vi "Begin.vi"(8 "error in":errorcluster) -> (0 "error out":errorcluster)   [LabVIEW 2017]
doc: "Called before other user functions, this VI is expected to open initial I/O refnums, load in file data, and do all program initialization. Notice that the <B>error out</B> terminal is simply used for data flow. Wiring it to other structures or subVIs ensures that this VI runs first."
uses:
  <vilib>/Rock Robotics/WPI/DriverStation/WPI_DriverStationRobotMode2.ctl
  <vilib>/Rock Robotics/WPI/Solenoid/WPI_SolenoidChannel.ctl
  <vilib>/Rock Robotics/WPI/ThirdParty/Phoenix-LabVIEW/Motor Controller/Controls/CTRE_Phoenix_MotorControl_NeutralMode.ctl
  <vilib>/Rock Robotics/SystemInterfaces/DIO/FPGA_DIOChannel.ctl
  <vilib>/Rock Robotics/WPI/Joystick/WPI_JoystickDeviceEnum.ctl
  <vilib>/Rock Robotics/WPI/ThirdParty/Phoenix-LabVIEW/Motor Controller/Controls/CTRE_Phoenix_MotorControl_VelocityMeasurementPeriod.ctl
  <vilib>/Rock Robotics/WPI/ThirdParty/Phoenix-LabVIEW/Motor Controller/Controls/CTRE_Phoenix_MotorControl_StatusFrameEnhanced.ctl
  Robot Global Data.vi
  <vilib>/Rock Robotics/WPI/Solenoid/WPI_SolenoidOpenDouble.vi
  <vilib>/Rock Robotics/WPI/Switch/WPI_SwitchOpenLimit.vi
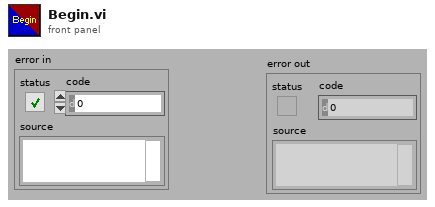
[diagram p1: front panel]
types:
  T1 = typedef "WPI_DriverStationRobotMode2.ctl" = enum16{"Autonomous Disabled", "Autonomous Enabled", "Teleop Disabled", "Teleop Enabled", "Disconnected", "Finish", "Test Disabled", "Test Enabled", "Emergency Stopped"}
  T2 = enum16{"Manual", "Turn For Angle", "Drive For Distance", "Motion Profile", "Recorded Auto File"}
  T3 = typedef "WPI_JoystickDeviceEnum.ctl" = enum16{"USB 0", "USB 1", "USB 2", "USB 3", "USB 4", "USB 5"}
  T4 = typedef "WPI_SolenoidChannel.ctl" = enum8{"Solenoid 0", "Solenoid 1", "Solenoid 2", "Solenoid 3", "Solenoid 4", "Solenoid 5", "Solenoid 6", "Solenoid 7", "Invalid"}
  T5 = typedef "CTRE_Phoenix_MotorControl_StatusFrameEnhanced.ctl" = u16
  T6 = typedef "CTRE_Phoenix_MotorControl_VelocityMeasurementPeriod.ctl" = u16
  T7 = typedef "WPI_MotorControlDeviceRef.ctl" = cluster{"DeviceStatus":errorcluster, "Type":T8, "PWM":cluster{"PWM Channel":T9, "DeadBand":T10}, "CAN":cluster{"Device Number":u8, "SetOutput VI Ref":variant, "GetOutput VI Ref":variant, "Enable VI Ref":variant, "Disable VI Ref":variant, "Data":variant}, "Invert":bool, "DIO PWM":cluster{"PWM \"Enable\" Channel":T9, "DIOChannel":T11, "PWM Rate":dbl}}
  T8 = typedef "WPI_MotorControlType.ctl" = enum16{"PWM", "CAN", "DIO PWM"}
  T9 = typedef "FPGA_DIOPWMChannel.ctl" = enum8{"PWM 0", "PWM 1", "PWM 2", "PWM 3", "PWM 4", "PWM 5", "PWM 6", "PWM 7", "PWM 8", "PWM 9", "PWM MXP 0", "PWM MXP 1", "PWM MXP 2", "PWM MXP 3", "PWM MXP 4", "PWM MXP 5", "PWM MXP 6", "PWM MXP 7", "PWM MXP 8", "PWM MXP 9", "Invalid"}
  T10 = typedef "WPI_PWMDeadband.ctl" = cluster{"Name":string, "maxPositivePwm":i32, "minPositivePwm":i32, "centerPwm":i32, "maxNegativePwm":i32, "minNegativePwm":i32, "angularRange":u16}
  T11 = typedef "FPGA_DIOChannel.ctl" = enum8{"DIO 0", "DIO 1", "DIO 2", "DIO 3", "DIO 4", "DIO 5", "DIO 6", "DIO 7", "DIO 8", "DIO 9", "DIO MXP 0", "DIO MXP 1", "DIO MXP 2", "DIO MXP 3", "DIO MXP 4", "DIO MXP 5", "DIO MXP 6", "DIO MXP 7", "DIO MXP 8", "DIO MXP 9", "DIO MXP 10", "DIO MXP 11", "DIO MXP 12", "DIO MXP 13", "DIO MXP 14", "DIO MXP 15", "SPI Port CS1", "SPI Port CS2", "SPI Port CS3", "SPI Port MISO", "SPI Port MOSI", "Invalid"}
  T12 = typedef "WPI_JoystickDevRef.ctl" = cluster{"Device":T3}
  T13 = typedef "WPI_SolenoidDevRef.ctl" = cluster{"DevStatus":errorcluster, "Pneumatics Control Module":u8, "Forward Solenoid Channel":T4, "Reverse Solenoid Channel":T4}
  T14 = typedef "CTRE_Phoenix_MotorControl_NeutralMode.ctl" = enum8{"EEPROMSetting", "Override to Coast", "Override to Brake"}
  T15 = typedef "WPI_SwitchDevRef.ctl" = cluster{"DevStatus":errorcluster, "DIO Channel":T11, "CntIndex":T16, "Normally Closed":bool}
  T16 = typedef "FPGA_CounterCtrSystemIndex.ctl" = enum8{"Ctr 0", "Ctr 1", "Ctr 2", "Ctr 3", "Ctr 4", "Ctr 5", "Ctr 6", "Ctr 7", "Invalid"}
  T17 = typedef "WPI_CompressorDevRef.ctl" = cluster{"DevStatus":errorcluster, "Pneumatics Control Module":u8}
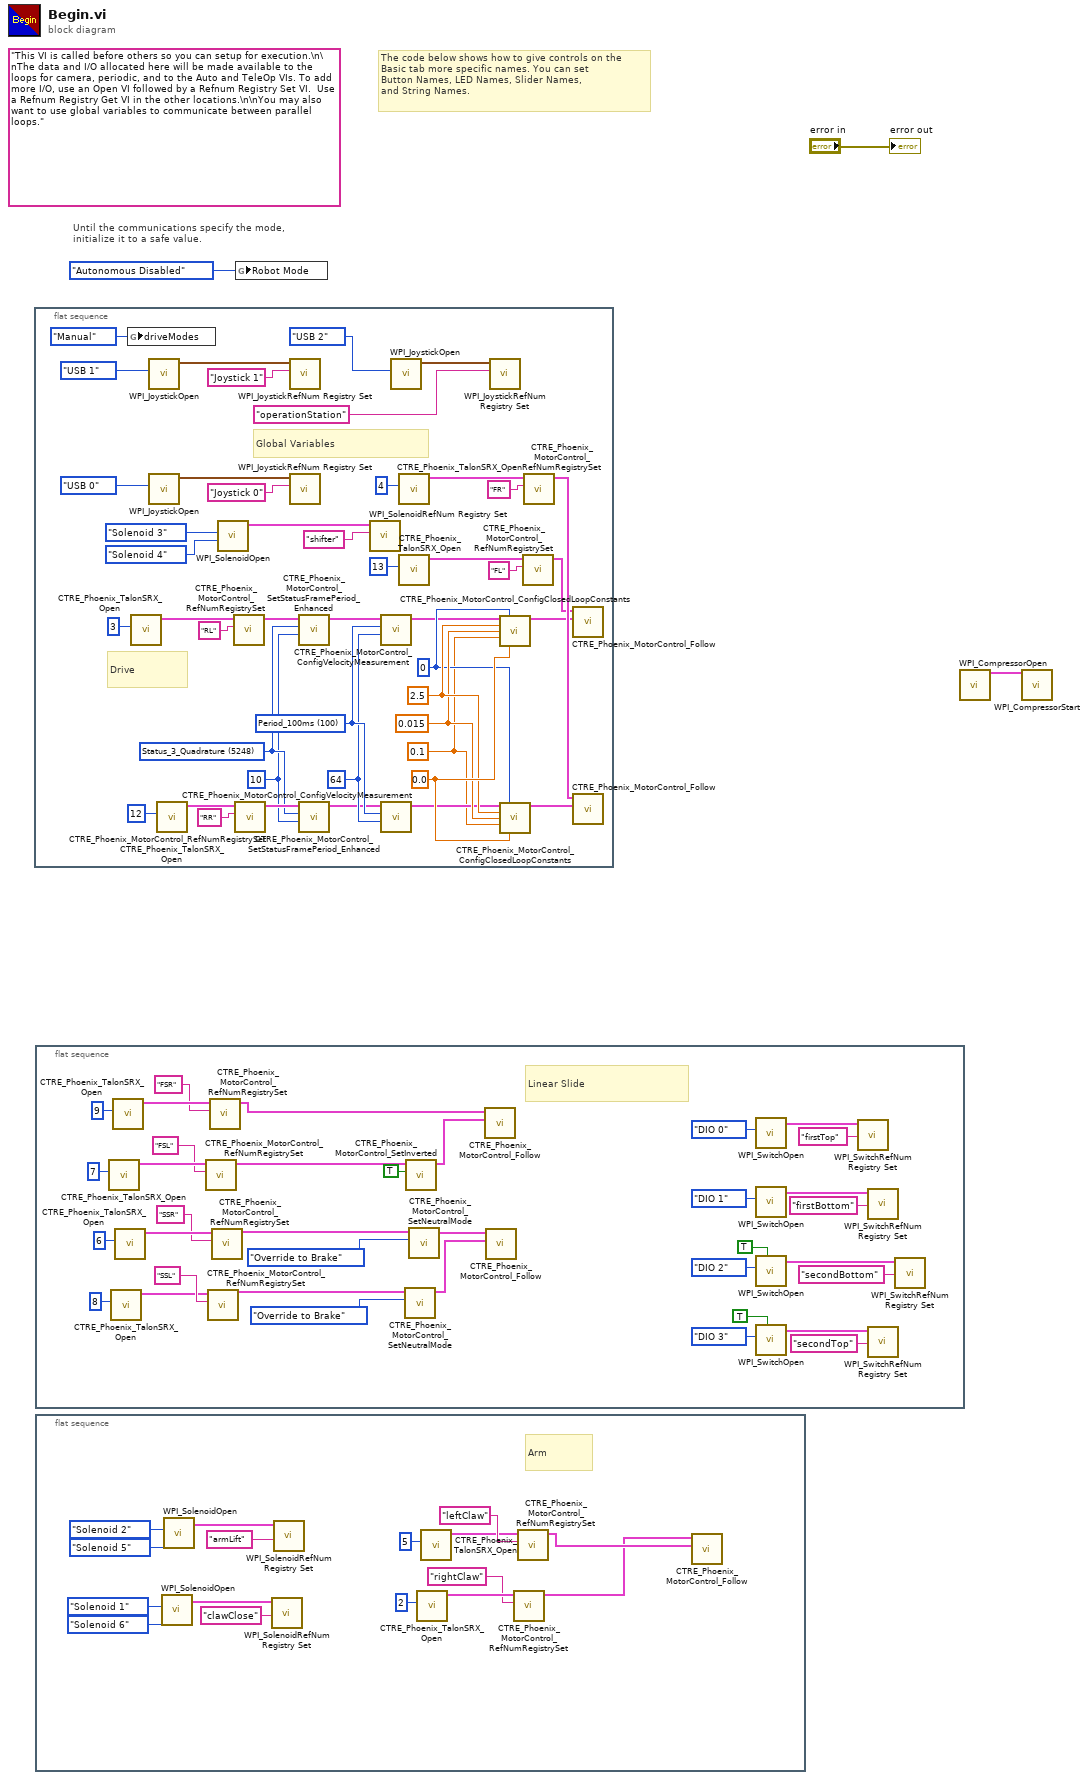
[diagram p0: block diagram]
diagram:
  (unwired) "This VI is called before others so you can setup for execution.\n\nThe data and I/O allocated here will be made available to the loops for camera, periodic, and to the Auto and TeleOp VIs. To add more I/O, use an Open VI followed by a Refnum Registry Set VI.  Use a Refnum Registry Get VI in the other locations.\n\nYou may also want to use global variables to communicate between parallel loops."
  # "The code below shows how to give controls on the\nBasic tab more specific names. You can set\nButton Names, LED Names, Slider Names,\nand String Names."
  # "Until the communications specify the mode,\ninitialize it to a safe value."
  n1 = flat-sequence {
    frame #0 {
      w4 = 10 ("periodMs")
      w5 = T5 5248 items=["Status_1_General"=5120, "Status_2_Feedback0"=5184, "Status_3_Quadrature"=5248, "Status_4_AinTempVbat"=5312, "Status_6_Misc"=5440, "Status_7_CommStatus"=5504, "Status_8_PulseWidth"=5568, "Status_9_MotProfBuffer"=5632, "Status_10_MotionMagic"=5696, "Status_11_UartGadgeteer"=5760, "Status_12_Feedback1"=5824, "Status_13_Base_PIDF0"=5888, "Status_14_Turn_PIDF1"=5952, "Status_15_FirmwareApiStatus"=6016] ("Status Frame")
      w11 = 0.1 ("D")
      w12 = 64 ("Window Size")
      w13 = T6 100 items=["Period_1ms"=1, "Period_2ms"=2, "Period_5ms"=5, "Period_10ms"=10, "Period_20ms"=20, "Period_25ms"=25, "Period_50ms"=50, "Period_100ms"=100] ("Velocity Measurement Period")
      w18 = 0.015 ("I")
      w19 = 2.5 ("P")
      w15 = 0 ("slotIdx")
      w20 = 0.0 ("F")
      # "Global Variables"
      # "Drive"
      n2 = global write "Robot Global Data.vi" "driveModes"(T2."Manual" ("driveModes")) -> ()
      n3 = call <vilib>:"CTRE_Phoenix_TalonSRX_Open.vi"("Device Number"=u8 3) -> ("CAN Talon SRX Ref"=w37:T7)  [unwired: 9 in, 1 out]
      n4 = call <vilib>:"WPI_JoystickOpen.vi"("JoystickDevice"=WPI_JoystickDeviceEnum."USB 1") -> ("JoystickDevRef"=w47:T12)  [unwired: 10 in]
      n5 = call <vilib>:"WPI_JoystickOpen.vi"("JoystickDevice"=WPI_JoystickDeviceEnum."USB 0") -> ("JoystickDevRef"=w44:T12)  [unwired: 10 in]
      n6 = call <vilib>:"CTRE_Phoenix_TalonSRX_Open.vi"("Device Number"=u8 12) -> ("CAN Talon SRX Ref"=w31:T7)  [unwired: 9 in, 1 out]
      n7 = call-poly <vilib>:"WPI_SolenoidOpen.vi"("Reverse Solenoid Channel"=WPI_SolenoidChannel."Solenoid 4", "Forward Solenoid Channel"=WPI_SolenoidChannel."Solenoid 3") -> ("SolenoidDevRef"=w30:T13)  [unwired: 8 in, 1 out]
      n8 = call <vilib>:"CTRE_Phoenix_MotorControl_RefNumRegistrySet.vi"("refnum name"="RL", "PhoenixMotorControlDevRef"=w37) -> ("PhoenixMotorControlDevRef"=w9:T7)  [unwired: 8 in, 1 out]
      n9 = call <vilib>:"CTRE_Phoenix_MotorControl_RefNumRegistrySet.vi"("refnum name"="RR", "PhoenixMotorControlDevRef"=w31) -> ("PhoenixMotorControlDevRef"=w7:T7)  [unwired: 8 in, 1 out]
      n10 = call <vilib>:"WPI_JoystickRefNum Registry Set.vi"("refnum name"="Joystick 1", "JoystickDevRef"=w47) -> ()  [unwired: 8 in, 2 out]
      n11 = call <vilib>:"WPI_JoystickRefNum Registry Set.vi"("refnum name"="Joystick 0", "JoystickDevRef"=w44) -> ()  [unwired: 8 in, 2 out]
      n12 = call <vilib>:"CTRE_Phoenix_MotorControl_SetStatusFramePeriod_Enhanced.vi"("periodMs"=w4, "Status Frame"=w5, "PhoenixMotorControlDevRef"=w9) -> ("PhoenixMotorControlDevRef"=w8:T7)  [unwired: 7 in, 1 out]
      n13 = call <vilib>:"CTRE_Phoenix_MotorControl_SetStatusFramePeriod_Enhanced.vi"("periodMs"=w4, "Status Frame"=w5, "PhoenixMotorControlDevRef"=w7) -> ("PhoenixMotorControlDevRef"=w6:T7)  [unwired: 7 in, 1 out]
      n14 = call <vilib>:"WPI_SolenoidRefNum Registry Set.vi"("refnum name"="shifter", "SolenoidDevRef"=w30) -> ()  [unwired: 8 in, 2 out]
      n15 = call <vilib>:"CTRE_Phoenix_MotorControl_ConfigVelocityMeasurement.vi"("Window Size"=w12, "Velocity Measurement Period"=w13, "PhoenixMotorControlDevRef"=w8) -> ("PhoenixMotorControlDevRef"=w14:T7)  [unwired: 7 in, 1 out]
      n16 = call <vilib>:"CTRE_Phoenix_MotorControl_ConfigVelocityMeasurement.vi"("Window Size"=w12, "Velocity Measurement Period"=w13, "PhoenixMotorControlDevRef"=w6) -> ("PhoenixMotorControlDevRef"=w16:T7)  [unwired: 7 in, 1 out]
      n17 = call <vilib>:"WPI_JoystickOpen.vi"("JoystickDevice"=WPI_JoystickDeviceEnum."USB 2") -> ("JoystickDevRef"=w25:T12)  [unwired: 10 in]
      n18 = call <vilib>:"CTRE_Phoenix_TalonSRX_Open.vi"("Device Number"=u8 4) -> ("CAN Talon SRX Ref"=w36:T7)  [unwired: 9 in, 1 out]
      n19 = call <vilib>:"CTRE_Phoenix_TalonSRX_Open.vi"("Device Number"=u8 13) -> ("CAN Talon SRX Ref"=w42:T7)  [unwired: 9 in, 1 out]
      n20 = call <vilib>:"WPI_JoystickRefNum Registry Set.vi"("refnum name"="operationStation", "JoystickDevRef"=w25) -> ()  [unwired: 8 in, 2 out]
      n21 = call <vilib>:"CTRE_Phoenix_MotorControl_ConfigClosedLoopConstants.vi"("PhoenixMotorControlDevRef"=w14, "slotIdx"=w15, "P"=w19, "I"=w18, "D"=w11, "F"=w20) -> ("PhoenixMotorControlDevRef"=w21:T7)  [unwired: 8 in, 1 out]
      n22 = call <vilib>:"CTRE_Phoenix_MotorControl_ConfigClosedLoopConstants.vi"("PhoenixMotorControlDevRef"=w16, "slotIdx"=w15, "P"=w19, "I"=w18, "D"=w11, "F"=w20) -> ("PhoenixMotorControlDevRef"=w17:T7)  [unwired: 8 in, 1 out]
      n23 = call <vilib>:"CTRE_Phoenix_MotorControl_RefNumRegistrySet.vi"("refnum name"="FL", "PhoenixMotorControlDevRef"=w42) -> ("PhoenixMotorControlDevRef"=w22:T7)  [unwired: 8 in, 1 out]
      n24 = call <vilib>:"CTRE_Phoenix_MotorControl_RefNumRegistrySet.vi"("refnum name"="FR", "PhoenixMotorControlDevRef"=w36) -> ("PhoenixMotorControlDevRef"=w23:T7)  [unwired: 8 in, 1 out]
      n25 = call <vilib>:"CTRE_Phoenix_MotorControl_Follow.vi"("Master Controller to Follow"=w21, "PhoenixMotorControlDevRef"=w22) -> ()  [unwired: 8 in, 2 out]
      n26 = call <vilib>:"CTRE_Phoenix_MotorControl_Follow.vi"("Master Controller to Follow"=w17, "PhoenixMotorControlDevRef"=w23) -> ()  [unwired: 8 in, 2 out]
    }
  }
  n27 = flat-sequence {
    frame #0 {
      # "Linear Slide"
      n28 = call <vilib>:"CTRE_Phoenix_TalonSRX_Open.vi"("Device Number"=u8 7) -> ("CAN Talon SRX Ref"=w84:T7)  [unwired: 9 in, 1 out]
      n29 = call <vilib>:"CTRE_Phoenix_TalonSRX_Open.vi"("Device Number"=u8 8) -> ("CAN Talon SRX Ref"=w70:T7)  [unwired: 9 in, 1 out]
      n30 = call <vilib>:"CTRE_Phoenix_TalonSRX_Open.vi"("Device Number"=u8 9) -> ("CAN Talon SRX Ref"=w80:T7)  [unwired: 9 in, 1 out]
      n31 = call <vilib>:"CTRE_Phoenix_TalonSRX_Open.vi"("Device Number"=u8 6) -> ("CAN Talon SRX Ref"=w74:T7)  [unwired: 9 in, 1 out]
      n32 = call <vilib>:"CTRE_Phoenix_MotorControl_RefNumRegistrySet.vi"("refnum name"="FSL", "PhoenixMotorControlDevRef"=w84) -> ("PhoenixMotorControlDevRef"=w77:T7)  [unwired: 8 in, 1 out]
      n33 = call <vilib>:"CTRE_Phoenix_MotorControl_RefNumRegistrySet.vi"("refnum name"="SSL", "PhoenixMotorControlDevRef"=w70) -> ("PhoenixMotorControlDevRef"=w76:T7)  [unwired: 8 in, 1 out]
      n34 = call <vilib>:"CTRE_Phoenix_MotorControl_RefNumRegistrySet.vi"("refnum name"="FSR", "PhoenixMotorControlDevRef"=w80) -> ("PhoenixMotorControlDevRef"=w78:T7)  [unwired: 8 in, 1 out]
      n35 = call <vilib>:"CTRE_Phoenix_MotorControl_RefNumRegistrySet.vi"("refnum name"="SSR", "PhoenixMotorControlDevRef"=w74) -> ("PhoenixMotorControlDevRef"=w75:T7)  [unwired: 8 in, 1 out]
      n36 = call <vilib>:"CTRE_Phoenix_MotorControl_SetNeutralMode.vi"("Motor Control Neutral Mode"=CTRE_Phoenix_MotorControl_NeutralMode."Override to Brake", "PhoenixMotorControlDevRef"=w76) -> ("PhoenixMotorControlDevRef"=w65:T7)  [unwired: 8 in, 1 out]
      n37 = call <vilib>:"CTRE_Phoenix_MotorControl_SetInverted.vi"("Invert?"=TRUE, "PhoenixMotorControlDevRef"=w77) -> ("PhoenixMotorControlDevRef"=w68:T7)  [unwired: 8 in, 1 out]
      n38 = call <vilib>:"CTRE_Phoenix_MotorControl_SetNeutralMode.vi"("Motor Control Neutral Mode"=CTRE_Phoenix_MotorControl_NeutralMode."Override to Brake", "PhoenixMotorControlDevRef"=w75) -> ("PhoenixMotorControlDevRef"=w66:T7)  [unwired: 8 in, 1 out]
      n39 = call <vilib>:"CTRE_Phoenix_MotorControl_Follow.vi"("Master Controller to Follow"=w68, "PhoenixMotorControlDevRef"=w78) -> ()  [unwired: 8 in, 2 out]
      n40 = call <vilib>:"CTRE_Phoenix_MotorControl_Follow.vi"("Master Controller to Follow"=w65, "PhoenixMotorControlDevRef"=w66) -> ()  [unwired: 8 in, 2 out]
      n41 = call-poly <vilib>:"WPI_SwitchOpen.vi"("DIO Channel"=FPGA_DIOChannel."DIO 0") -> ("SwitchDevRef"=w61:T15)  [unwired: 9 in, 1 out]
      n42 = call-poly <vilib>:"WPI_SwitchOpen.vi"("DIO Channel"=FPGA_DIOChannel."DIO 1") -> ("SwitchDevRef"=w58:T15)  [unwired: 9 in, 1 out]
      n43 = call-poly <vilib>:"WPI_SwitchOpen.vi"("Normally Closed"=TRUE, "DIO Channel"=FPGA_DIOChannel."DIO 2") -> ("SwitchDevRef"=w52:T15)  [unwired: 8 in, 1 out]
      n44 = call-poly <vilib>:"WPI_SwitchOpen.vi"("Normally Closed"=TRUE, "DIO Channel"=FPGA_DIOChannel."DIO 3") -> ("SwitchDevRef"=w55:T15)  [unwired: 8 in, 1 out]
      n45 = call <vilib>:"WPI_SwitchRefNum Registry Set.vi"("refnum name"="firstTop", "SwitchDevRef"=w61) -> ()  [unwired: 8 in, 2 out]
      n46 = call <vilib>:"WPI_SwitchRefNum Registry Set.vi"("refnum name"="firstBottom", "SwitchDevRef"=w58) -> ()  [unwired: 8 in, 2 out]
      n47 = call <vilib>:"WPI_SwitchRefNum Registry Set.vi"("refnum name"="secondTop", "SwitchDevRef"=w55) -> ()  [unwired: 8 in, 2 out]
      n48 = call <vilib>:"WPI_SwitchRefNum Registry Set.vi"("refnum name"="secondBottom", "SwitchDevRef"=w52) -> ()  [unwired: 8 in, 2 out]
    }
  }
  n49 = flat-sequence {
    frame #0 {
      # "Arm"
      n50 = call-poly <vilib>:"WPI_SolenoidOpen.vi"("Reverse Solenoid Channel"=WPI_SolenoidChannel."Solenoid 6", "Forward Solenoid Channel"=WPI_SolenoidChannel."Solenoid 1") -> ("SolenoidDevRef"=w96:T13)  [unwired: 8 in, 1 out]
      n51 = call-poly <vilib>:"WPI_SolenoidOpen.vi"("Reverse Solenoid Channel"=WPI_SolenoidChannel."Solenoid 5", "Forward Solenoid Channel"=WPI_SolenoidChannel."Solenoid 2") -> ("SolenoidDevRef"=w97:T13)  [unwired: 8 in, 1 out]
      n52 = call <vilib>:"WPI_SolenoidRefNum Registry Set.vi"("refnum name"="clawClose", "SolenoidDevRef"=w96) -> ()  [unwired: 8 in, 2 out]
      n53 = call <vilib>:"WPI_SolenoidRefNum Registry Set.vi"("refnum name"="armLift", "SolenoidDevRef"=w97) -> ()  [unwired: 8 in, 2 out]
      n54 = call <vilib>:"CTRE_Phoenix_TalonSRX_Open.vi"("Device Number"=u8 2) -> ("CAN Talon SRX Ref"=w91:T7)  [unwired: 9 in, 1 out]
      n55 = call <vilib>:"CTRE_Phoenix_TalonSRX_Open.vi"("Device Number"=u8 5) -> ("CAN Talon SRX Ref"=w87:T7)  [unwired: 9 in, 1 out]
      n56 = call <vilib>:"CTRE_Phoenix_MotorControl_RefNumRegistrySet.vi"("refnum name"="rightClaw", "PhoenixMotorControlDevRef"=w91) -> ("PhoenixMotorControlDevRef"=w85:T7)  [unwired: 8 in, 1 out]
      n57 = call <vilib>:"CTRE_Phoenix_MotorControl_RefNumRegistrySet.vi"("refnum name"="leftClaw", "PhoenixMotorControlDevRef"=w87) -> ("PhoenixMotorControlDevRef"=w86:T7)  [unwired: 8 in, 1 out]
      n58 = call <vilib>:"CTRE_Phoenix_MotorControl_Follow.vi"("Master Controller to Follow"=w86, "PhoenixMotorControlDevRef"=w85) -> ()  [unwired: 8 in, 2 out]
    }
  }
  n59 = global write "Robot Global Data.vi" "Robot Mode"(WPI_DriverStationRobotMode2."Autonomous Disabled" ("Robot Mode")) -> ()
  n60 = call <vilib>:"WPI_CompressorOpen.vi"() -> ("CompressorDevRef"=w1:T17)  [unwired: 14 in, 1 out]
  n61 = call <vilib>:"WPI_CompressorStart.vi"("CompressorDevRef"=w1) -> ()  [unwired: 9 in, 2 out]
  "error out" <- "error in"
